vi "CalculateCI.vi"(8 "k degrees of freedom (n-1)":i32=1, 9 "Confidence Level":dbl, 10 "Standard Deviation":dbl, 11 "Mean":dbl) -> (0 "low":dbl, 1 "high":dbl, 2 "Width":dbl)   [LabVIEW 2013]
doc: "This VI calculates confidence intervals (based on inverse Student's t-distribution), given mean, stdev, and degrees of freedom (i.e., number of samples - 1)."
uses:
  <vilib>/gmath/statdist.llb/Student t Inverse CDF.vi
  <vilib>/gmath/NI_Gmath.lvlib
panel:
  # "This SubVI calculates confidence intervals given mean, standard deviation, and degrees of freedom (i.e., number of samples - 1)."
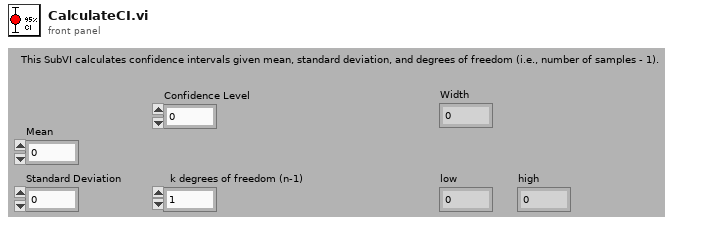
[diagram p1: front panel]
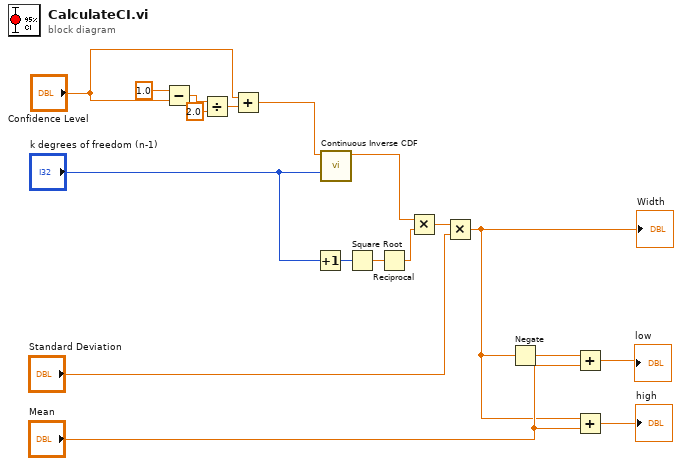
[diagram p0: block diagram]
diagram:
  n1 = Subtract(x=1.0, y="Confidence Level") -> (x-y=w17:dbl)
  n2 = Divide(x=w17, y=2.0) -> (x/y=w15:dbl)
  n3 = Add(x="Confidence Level", y=w15) -> (x+y=w13:dbl)
  n4 = Increment(x="k degrees of freedom (n-1)") -> (x+1=w12:i32)
  n5 = call-poly <vilib>:"Continuous Inverse CDF.vi"("k degrees of freedom"="k degrees of freedom (n-1)", "cdf(x)"=w13) -> ("x"=w8:dbl)  [unwired: 8 in, 1 out]
  n6 = Square Root(x=w12) -> (sqrt(x)=w11:dbl)
  n7 = Reciprocal(x=w11) -> (1/x=w9:dbl)
  n8 = Multiply(x=w8, y=w9) -> (x*y=w7:dbl)
  n9 = Multiply(x=w7, y="Standard Deviation") -> (x*y=w1:dbl)
  "Width" <- w1
  n10 = Negate(x=w1) -> (-x=w3:dbl)
  n11 = Add(x=w3, y="Mean") -> (x+y=→"low":dbl)
  n12 = Add(x=w1, y="Mean") -> (x+y=→"high":dbl)
